vi "Add Reference Control to Cluster and Rename.vi"(8 "error in (no error)":errorcluster, 9 "New Label.Text":string, 10 "Private Data Refs":T1, 11 "GObject in":refnum<vi>) -> (0 "error out":errorcluster, 3 "GObject out":refnum<vi>)   [LabVIEW 2020, in "Add to Private Data.lvlib"]
uses:
  Add to Private Data.lvlib
  Private Data Refs.ctl
  <vilib>/Utility/miscctls.llb/LVPositionTypeDef.ctl
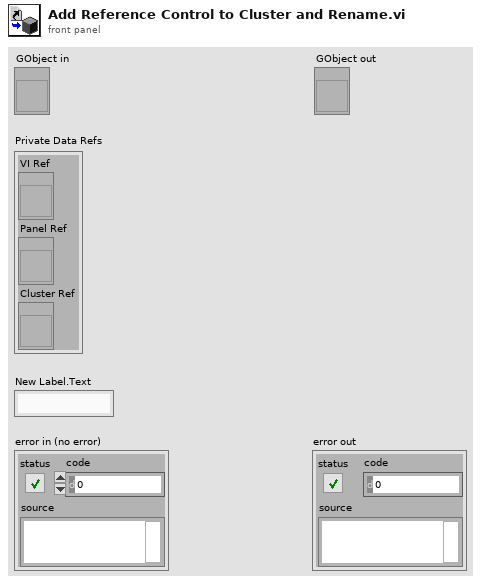
[diagram p1: front panel]
types:
  T1 = typedef "Add to Private Data.lvlib/Private Data Refs.ctl" = cluster{"VI Ref":refnum<vi>, "Panel Ref":refnum<vi>, "Cluster Ref":refnum<vi>}
  T2 = typedef "LVPositionTypeDef.ctl" = cluster{"Left":i32, "Top":i32}
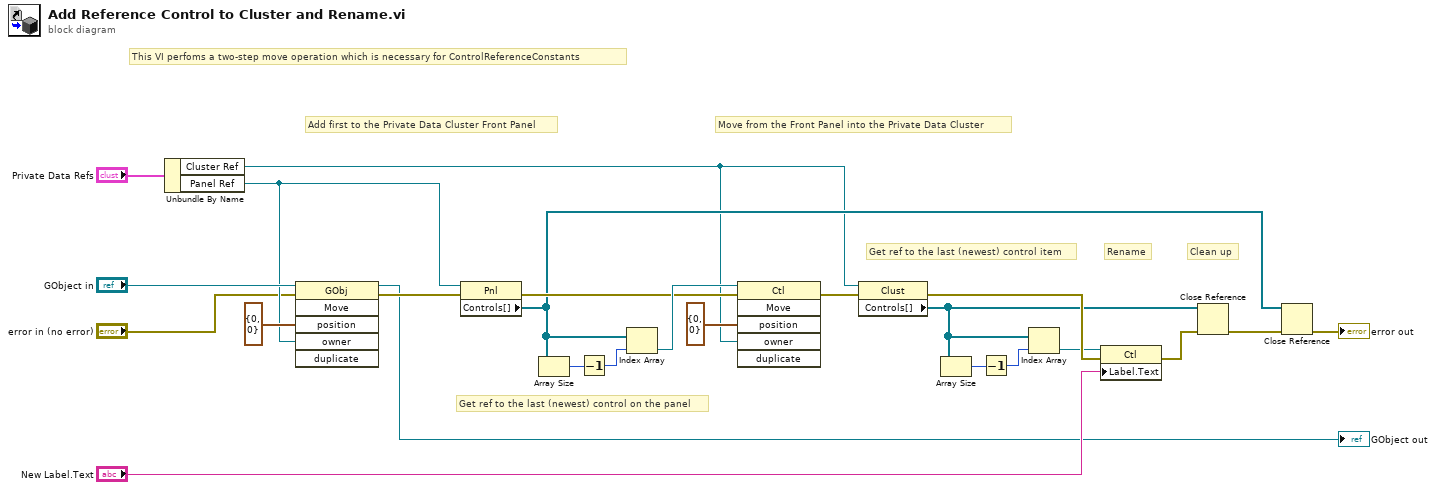
[diagram p0: block diagram]
diagram:
  # "This VI perfoms a two-step move operation which is necessary for ControlReferenceConstants"
  # "Move from the Front Panel into the Private Data Cluster"
  # "Add first to the Private Data Cluster Front Panel"
  # "Get ref to the last (newest) control on the panel"
  # "Clean up"
  # "Rename"
  # "Get ref to the last (newest) control item"
  n1 = Unbundle By Name("Private Data Refs") -> ("Cluster Ref"=w3:refnum<vi>, "Panel Ref"=w4:refnum<vi>)
  n2 = invoke class="GObj" method="Move"(reference="GObject in", error in="error in (no error)", "position"=T2 {"Left"=0, "Top"=0}, "owner"=w4) -> (reference out=→"GObject out":refnum<vi>, error out=w10:errorcluster)  [unwired: 2 in, 4 out]
  n3 = property class="Pnl"(reference=w4, error in=w10) -> (error out=w8:errorcluster, "Controls[]"=w6:refnum<vi>[])  [unwired: 1 out]
  n4 = Array Size(array=w6) -> (size(s)=w12:i32)
  n5 = Decrement(x=w12) -> (x-1=w11:i32)
  n6 = Index Array(array=w6, index=w11) -> (element=w9:refnum<vi>)
  n7 = invoke class="Ctl" method="Move"(reference=w9, error in=w8, "position"=T2 {"Left"=0, "Top"=0}, "owner"=w3) -> (error out=w22:errorcluster)  [unwired: 2 in, 5 out]
  n8 = property class="Clust"(reference=w3, error in=w22) -> (error out=w23:errorcluster, "Controls[]"=w18:refnum<vi>[])  [unwired: 1 out]
  n9 = Array Size(array=w18) -> (size(s)=w16:i32)
  n10 = Decrement(x=w16) -> (x-1=w17:i32)
  n11 = Index Array(array=w18, index=w17) -> (element=w19:refnum<vi>)
  n12 = property class="Ctl"(reference=w19, error in=w23, "Label.Text"="New Label.Text") -> (error out=w20:errorcluster)  [unwired: 1 out]
  n13 = Close Reference(reference=w18, error in (no error)=w20) -> (error out=w21:errorcluster)
  n14 = Close Reference(reference=w6, error in (no error)=w21) -> (error out=→"error out":errorcluster)
